vi "TFminiGet.vi"(11 "TFmini I2C DevRef":T1={"DevStatus"={"status"=FALSE, "code"=0, "source"=""}, "Device Address"=0, "Handle"=0, "I2C Bus"=enum."Invalid"} {"Device Address" format="%.0x"}) -> (1 "Raw (Inches)":dbl, 3 "Filtered (Inches)":dbl)   [LabVIEW 2018]
uses:
  <vilib>/Rock Robotics/WPI/I2C/WPI_I2CDevRef.ctl
  <vilib>/Rock Robotics/SystemInterfaces/i2clib/i2c_bus.ctl
panel:
  in  "hi limit":dbl=500.0 format="%#_13g"
  in  "lo limit":dbl format="%#_13g"
  out "Mode":bool=TRUE
  out "OOR":bool
  in  "Rate Thresh":dbl=700.0 step=0.001
  out "Strength":u16=120
  out "Distance (cm)":cluster{dbl, dbl, "Filtered":dbl}(graph)={34.25196850393701, 12.0, "Filtered"=34.25196850393701}
  out "Data Out":u8[](array[numeric])=[0, 87, 0, 120]
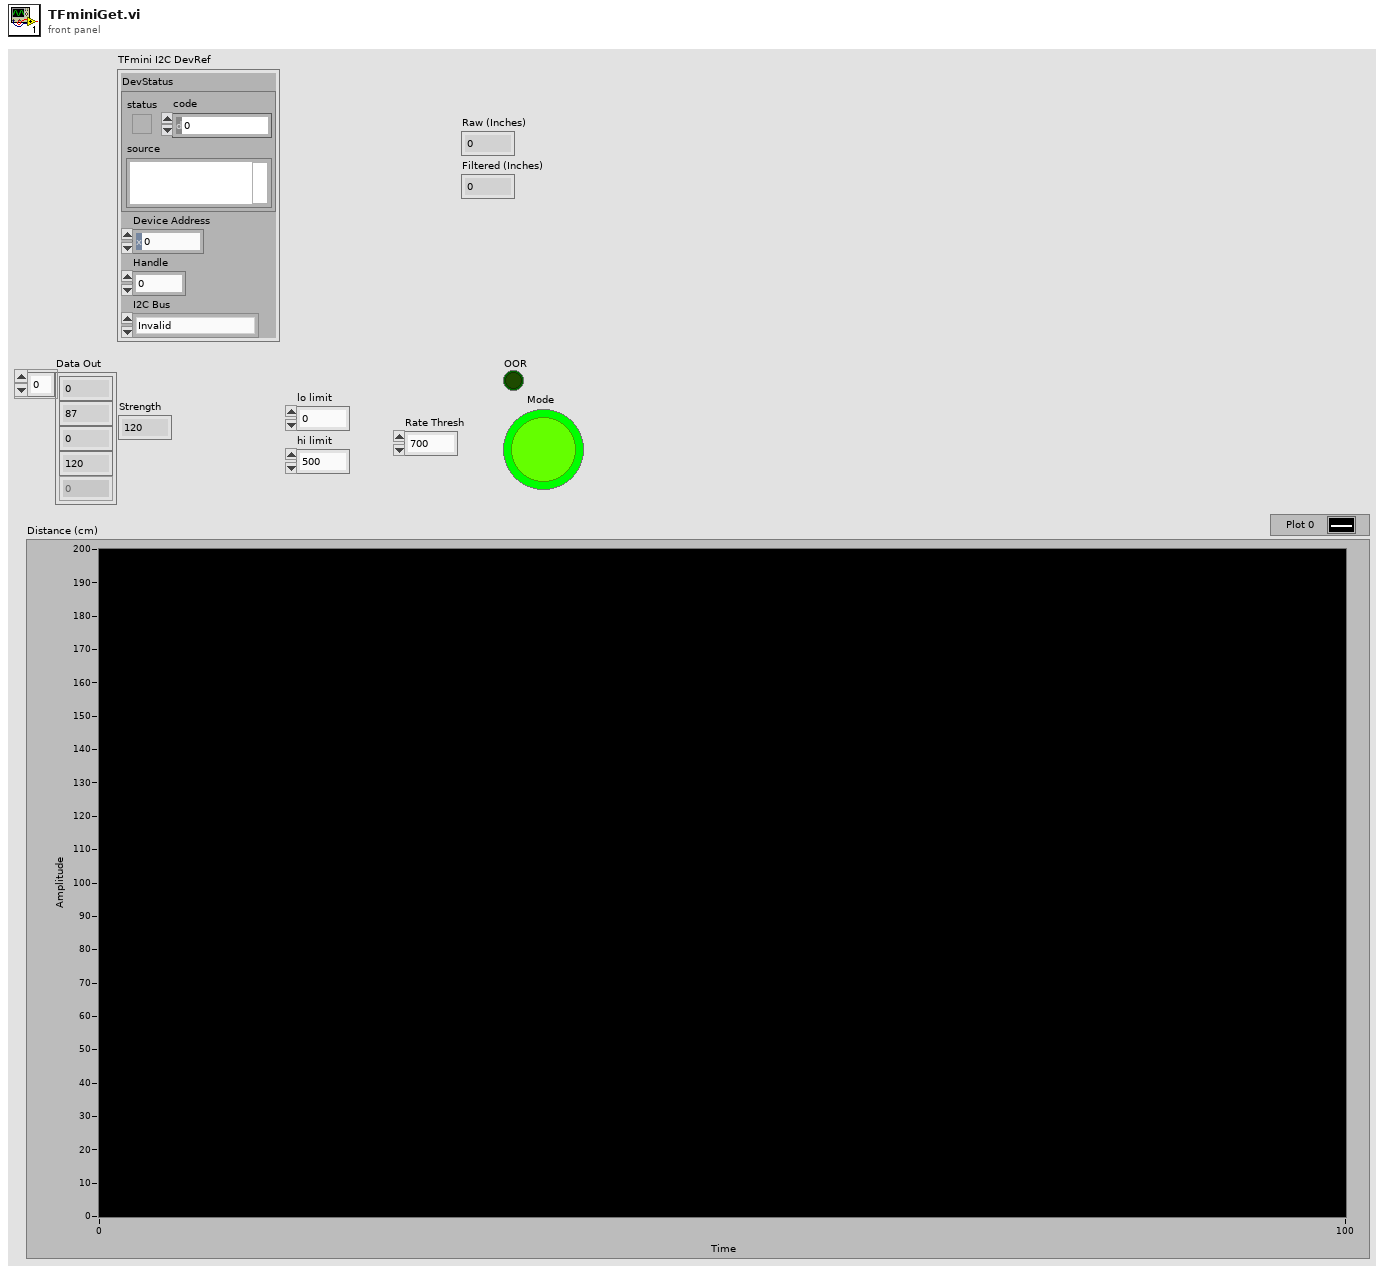
[diagram p1: front panel]
types:
  T1 = typedef "WPI_I2CDevRef.ctl" = cluster{"DevStatus":errorcluster, "Device Address":u8, "Handle":i32, "I2C Bus":T2}
  T2 = typedef "i2c_bus.ctl" = enum16{"I2C On-Board", "I2C MXP", "Invalid"}
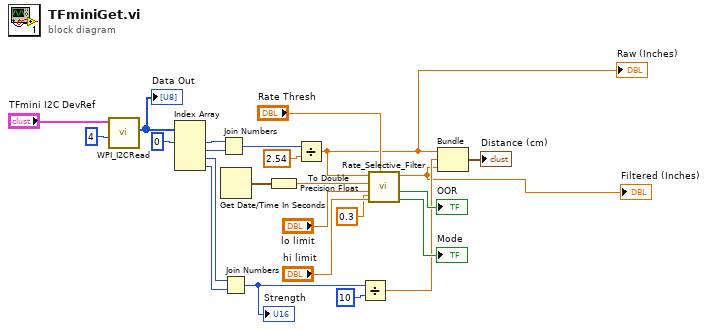
[diagram p0: block diagram]
diagram:
  n1 = call <vilib>:"WPI_I2CRead.vi"("I2CBytesToRead"=u8 4, "I2CDevRef"="TFmini I2C DevRef") -> ("Data Out"=w23:u8[])  [unwired: 7 in, 2 out]
  "Data Out" <- w23
  n2 = Index Array(array=w23, index #1=0 ("index")) -> (element #1=w21:u8, element #2=w20:u8, element #3=w19:u8, element #4=w18:u8)  [unwired: 3 in]
  n3 = Join Numbers(hi=w21, lo=w20) -> ((hi.lo)=w10:u16)
  n4 = Get Date/Time In Seconds() -> (seconds since 1Jan1904=w14:timestamp)
  n5 = Join Numbers(hi=w19, lo=w18) -> ((hi.lo)=w16:u16)
  "Strength" <- w16
  n6 = To Double Precision Float(number=w14) -> (double precision float=w13:dbl)
  n7 = Divide(x=w10, y=2.54) -> (x/y=w12:dbl)
  "Raw (Inches)" <- w12
  n8 = Divide(x=w16, y=u16 10) -> (x/y=w4:dbl)
  n9 = call <userlib>:"Rate_Selective_Filter.vi"("Hyster"=0.3, "Rate Thresh"="Rate Thresh", "hi limit"="hi limit", "lo limit"="lo limit", "Time"=w13, "Distance"=w12) -> ("Mode"=→"Mode":bool, "OOR"=→"OOR":bool, "Filtered"=w2:dbl)  [unwired: 1 in]
  "Filtered (Inches)" <- w2
  n10 = Bundle(w12, w4, "Filtered"=w2) -> (→"Distance (cm)":cluster{dbl, dbl, "Filtered":dbl})  [unwired: 1 in]
